vi "VrmVISACheckResponse.vi"(8 "error in (no error)":errorcluster, 10 "Response":string) -> (0 "error out":errorcluster, 2 "Response out":string)   [LabVIEW 2013]
uses:
  <vilib>/regexp/Match Regular Expression.xnode
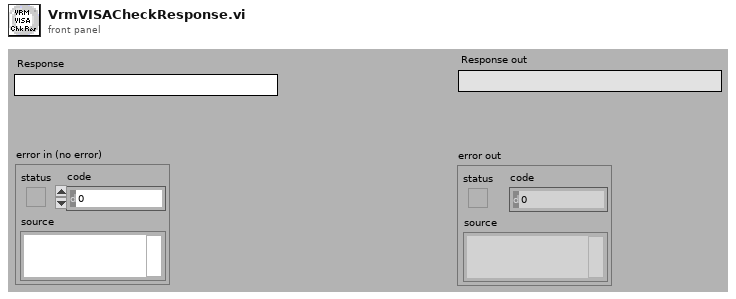
[diagram p1: front panel]
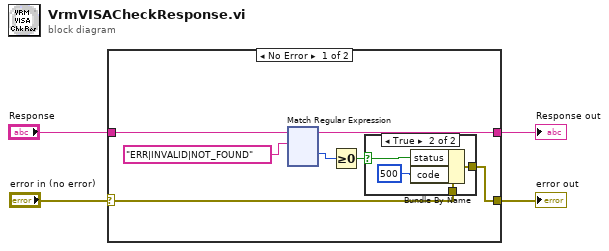
[diagram p0: block diagram]
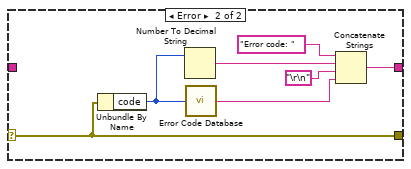
[diagram p3: hidden frame]
diagram:
  n1 = case shown="No Error" "error in (no error)" {
    selector: "error in (no error)" -> [w8 w133]
    tunnel: "Response" -> [w6 _]
    tunnel: [w9 w133] -> w2
    tunnel: [w6 w128] -> w1
    frame No Error {
      n2 = xnode "Match Regular Expression"("input string"=w6, "regular expression"="ERR|INVALID|NOT_FOUND") -> ("offset past match"=w7:i32)  [unwired: 4 in, 4 out]
      n3 = Greater Or Equal To 0?(x=w7) -> (x >= 0?=w5:bool)
      n4 = case shown="True" w5 {
        selector: w5 -> [_ w13]
        tunnel: [w11 w15] -> w9
        tunnel: w8 -> [w11 w14]
        frame False {
        }
        frame True {
          n5 = Bundle By Name(cluster=w14, "status"=w13, "code"=500) -> (w15:errorcluster)
        }
      }
    }
    frame Error {
      n6 = Unbundle By Name(w133) -> ("code"=w132:i32)
      n7 = Number To Decimal String(number=w132) -> (decimal integer string=w131:string)  [unwired: 1 in]
      n8 = call <vilib>:"Error Code Database.vi"("Error Code"=w132) -> ("Error Text"=w129:string)
      n9 = Concatenate Strings("Error code: " ("string"), w131, "\r\n", w129) -> (w128:string)
    }
  }
  "Response out" <- w1
  "error out" <- w2
